vi "Class Type Test.vi"() -> ()   [LabVIEW 2016, in "Better Search.lvlib" / "Search.lvclass"]
uses:
  Search.lvclass
  <vilib>/Utility/traverseref.llb/VI Scripting - Traverse.lvlib
  <vilib>/Utility/traverseref.llb/TRef TravTarget.ctl
  <vilib>/Utility/Data Type/NI_Data Type.lvlib
panel:
  out "VI Path":path
  out "error out":errorcluster
  out "Control VI Type":T1(ring)
  out "VI Type":T2(ring)
  out "Array":string[](array[string])
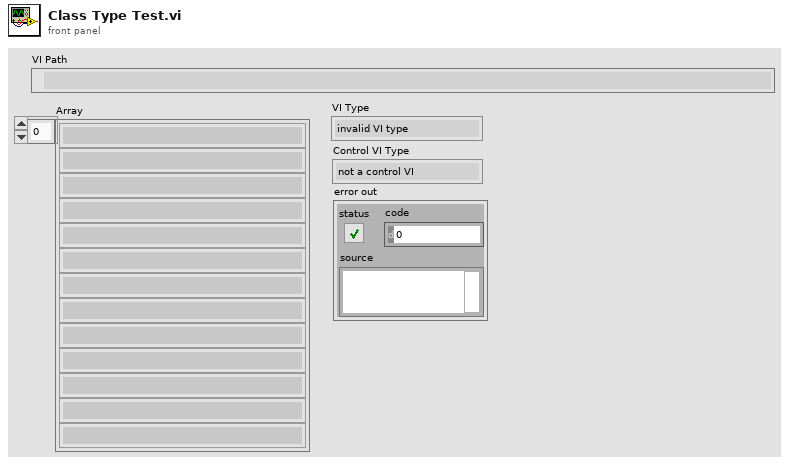
[diagram p1: front panel]
types:
  T1 = enum32{"not a control VI", "control", "typedef", "strict typedef"}
  T2 = enum32{"invalid VI type", "Standard VI", "Control VI", "Global VI", "Polymorphic VI", "Configuration VI", "SubSystem", "Facade VI", "Method VI", "Statechart Diagram VI"}
  T3 = typedef "TRef TravTarget.ctl" = enum16{"FP", "BD", "Other"}
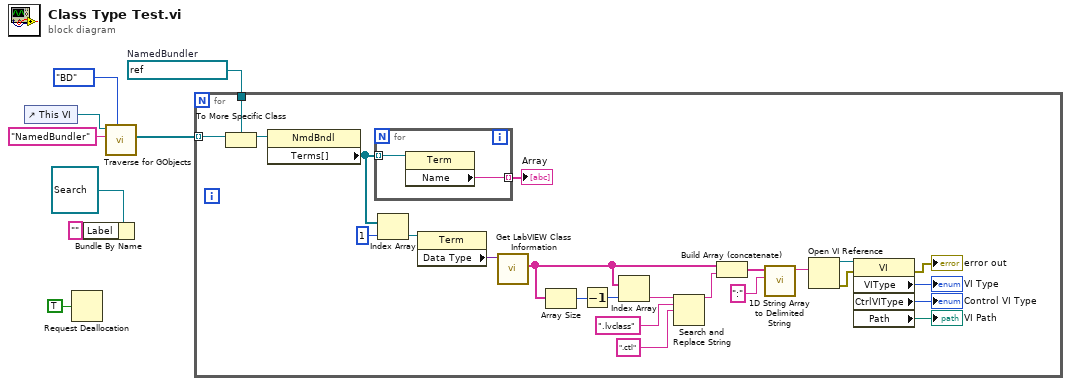
[diagram p0: block diagram]
diagram:
  w5 = refnum<vi> refnum  # NamedBundler
  n1 = control-ref of="This VI"() -> (w3:refnum<vi>)
  n2 = Request Deallocation(TRUE ("flag")) -> ()
  n3 = Bundle By Name(cluster=refnum<class "Search.lvclass"> refnum ("Better Search.lvlib:Search"), "Label"="" ("ID")) -> ()  [unwired: 1 out]
  n4 = call <vilib>:"Traverse for GObjects.vi"("Traverse Target"=TRef_TravTarget."BD", "Class Name"="NamedBundler", "VI Refnum"=w3) -> ("References"=w6:refnum<vi>[])  [unwired: 5 in, 3 out]
  n5 = for {
    tunnel: w6 -> [w32] mode=indexing
    tunnel: w5 -> [w31]
    n6 = To More Specific Class(target class=w31, reference=w32) -> (specific class reference=w30:refnum<vi>)  [unwired: 1 in, 1 out]
    n7 = property class="NmdBndl"(reference=w30) -> ("Terms[]"=w28:refnum<vi>[])  [unwired: 1 in, 2 out]
    n8 = for {
      tunnel: w28 -> [w34] mode=indexing
      tunnel: [w33] -> w29 mode=indexing
      n9 = property class="Term"(reference=w34) -> ("Name"=w33:string)  [unwired: 1 in, 2 out]
    }
    "Array" <- w29
    n10 = Index Array(array=w28, index=1) -> (element=w26:refnum<vi>)
    n11 = property class="Term"(reference=w26) -> ("Data Type"=w25:variant)  [unwired: 1 in, 2 out]
    n12 = call <vilib>:"Get LabVIEW Class Information.vi"("variant"=w25) -> ("qualified LabVIEW class name"=w21:string[])  [unwired: 8 in, 2 out]
    n13 = Array Size(array=w21) -> (size(s)=w23:i32)
    n14 = Decrement(x=w23) -> (x-1=w22:i32)
    n15 = Index Array(array=w21, index=w22) -> (element=w20:string)
    n16 = Search and Replace String(input string=w20, search string=".lvclass", replace string=".ctl" ("search string")) -> (result string=w17:string)  [unwired: 5 in, 3 out]
    n17 = Build Array (concatenate)(w21, w17) -> (w16:string[])
    n18 = call <vilib>:"1D String Array to Delimited String.vi"("delimiter"=":", "string array"=w16) -> ("delimited string"=w15:string)  [unwired: 9 in]
    n19 = Open VI Reference(vi path=w15) -> (vi reference=w14:refnum<vi>, error out=w12:errorcluster)  [unwired: 5 in]
    n20 = property class="VI"(reference=w14, error in=w12) -> (error out=→"error out":errorcluster, "VIType"=→"VI Type":T2, "CtrlVIType"=→"Control VI Type":T1, "Path"=→"VI Path":path)  [unwired: 1 out]
  }
